vi "Read stage position (set) [fs].vi"(8 "error in (no error)":errorcluster, 11 "_data in":refnum<class "_data.lvclass">) -> (0 "error out":errorcluster, 2 "stage position (set) [fs]":dbl[](array[numeric]), 3 "_data out":refnum<class "_data.lvclass">)   [LabVIEW 2019, in "_data.lvlib" / "_data.lvclass"]
uses:
  _data.lvclass
  _data.lvclass/_data.ctl
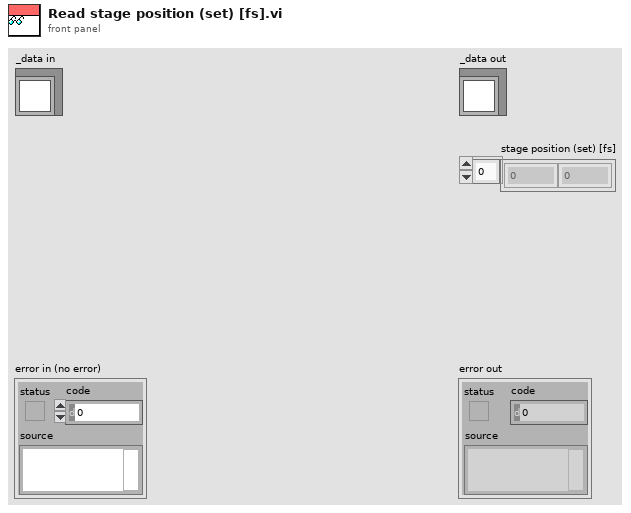
[diagram p1: front panel]
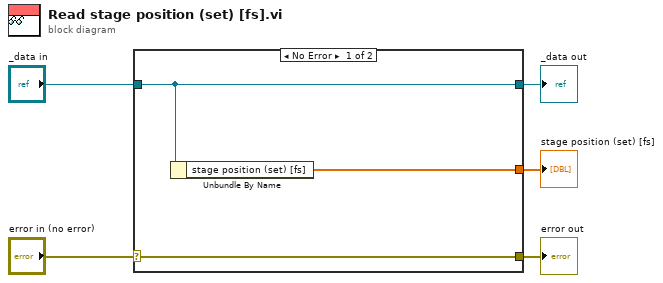
[diagram p0: block diagram]
diagram:
  n1 = case shown="No Error" "error in (no error)" {
    selector: "error in (no error)" -> [w8 w9]
    tunnel: [w8 w9] -> w4
    tunnel: [w7 w10] -> w2
    tunnel: "_data in" -> [w7 w10]
    tunnel: [w6 _] -> w1
    frame No Error {
      n2 = Unbundle By Name(w7) -> ("stage position (set) [fs]"=w6:dbl[])
    }
    frame Error {
    }
  }
  "error out" <- w4
  "_data out" <- w2
  "stage position (set) [fs]" <- w1
